vi "Choose case dewbot 10.vi"(4 "Next FR motor value":dbl=0.6, 6 "Next BL motor value":dbl=0.6, 9 "Next BR motor value":dbl=0.6, 10 "Next FL motor value":dbl=0.6, 11 "Set Tac value":dbl) -> (0 "Last FR motor value":dbl=0.6, 1 "Last BL motor value":dbl=0.6, 2 "Last BR motor value":dbl=0.6, 3 "Last FL motor value":dbl=0.6, 5 "Next primitive?":bool)   [LabVIEW 2013]
uses:
  Begin/Global Variables.vi
  Begin/Global Refnums.vi
  <vilib>/Rock Robotics/WPI/DriverStation/DriverStationLCD/WPI_DriverStationLCDLCDLine.ctl
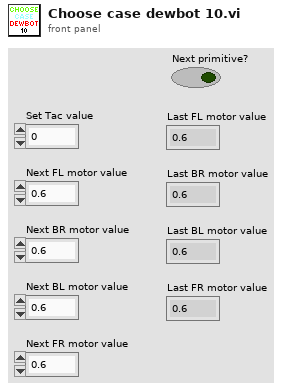
[diagram p1: front panel]
types:
  T1 = typedef "WPI_DriverStationLCDLCDLine.ctl" = enum16{"Main - Line 1", "User - Line 2", "User - Line 3", "User - Line 4", "User - Line 5", "User - Line 6"}
  T2 = typedef "WPI_GyroDevRef.ctl" = cluster{"DevStatus":errorcluster, "Analog Module":T3, "Analog Channel":T4, "Offset":dbl, "Gain (VoltsPerDegree/Second)":dbl}
  T3 = typedef "FPGA_TypedefAnalogModule.ctl" = enum16{"Analog Module 1", "Analog Module 2"}
  T4 = typedef "FPGA_AIChannel.ctl" = enum8{"AI 1", "AI 2", "AI 3", "AI 4", "AI 5", "AI 6", "AI 7", "AI 8", "Invalid"}
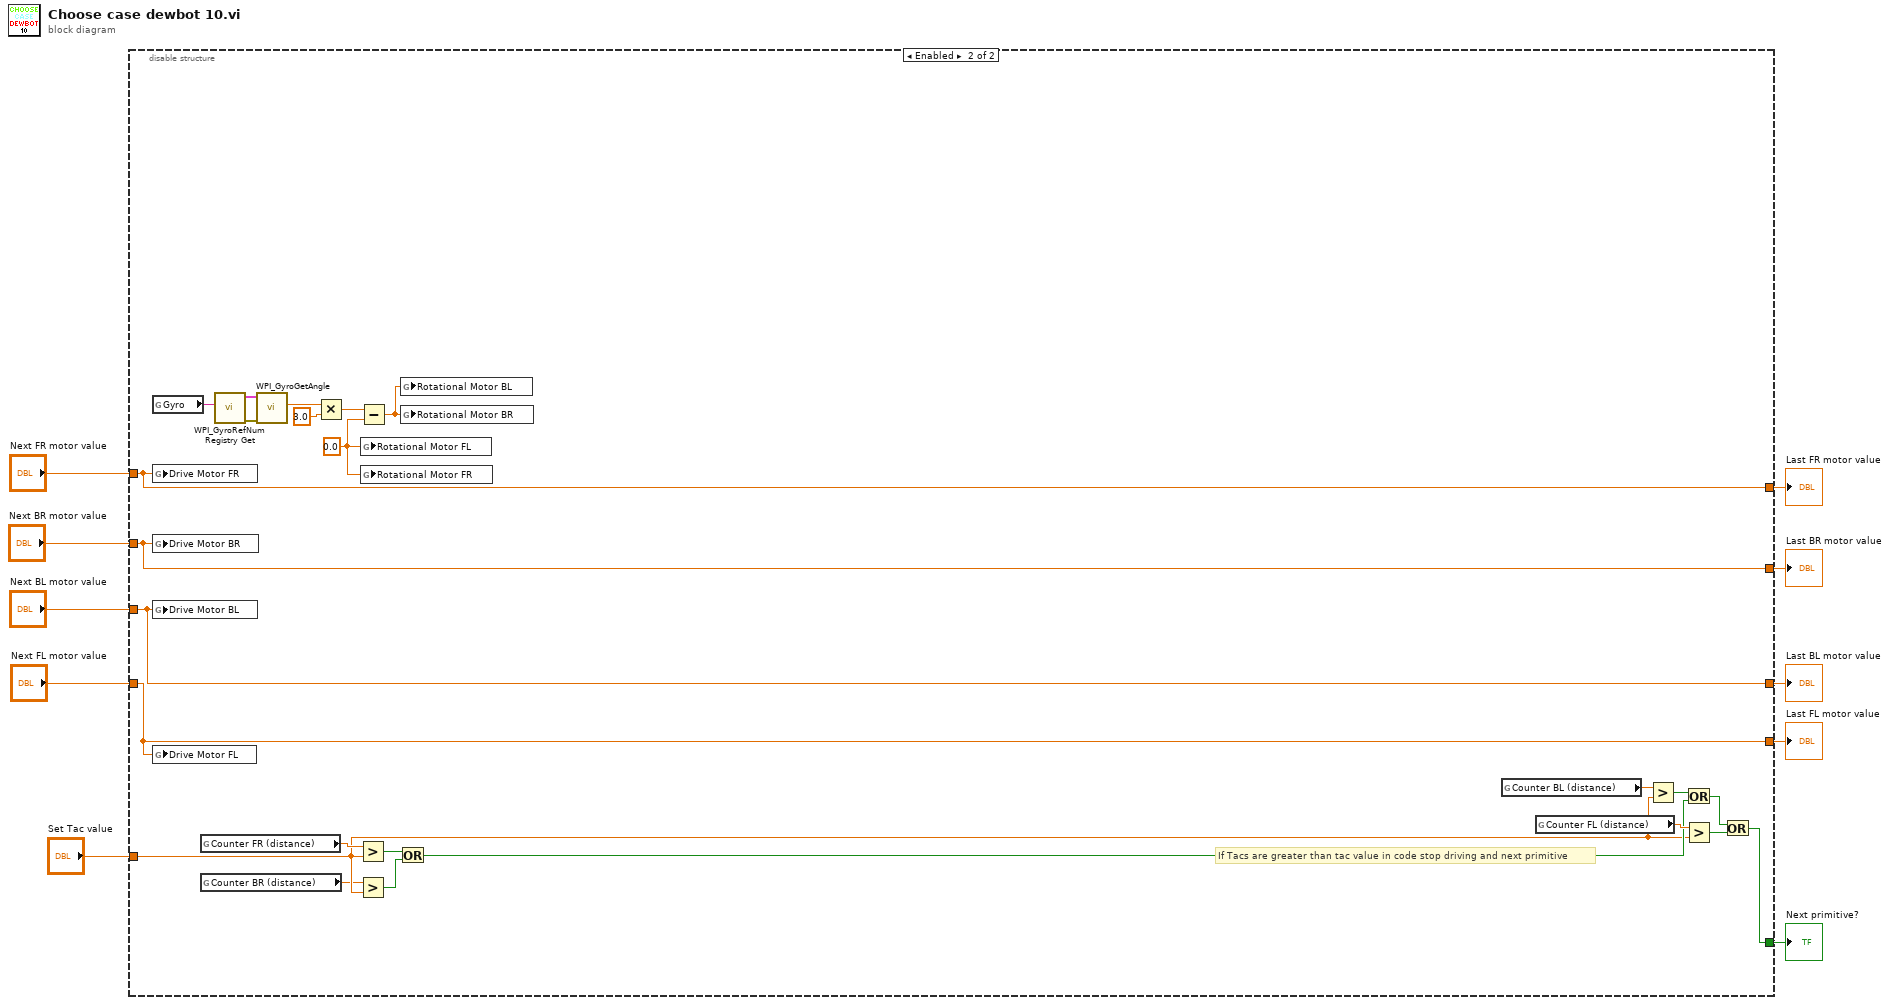
[diagram p0: block diagram]
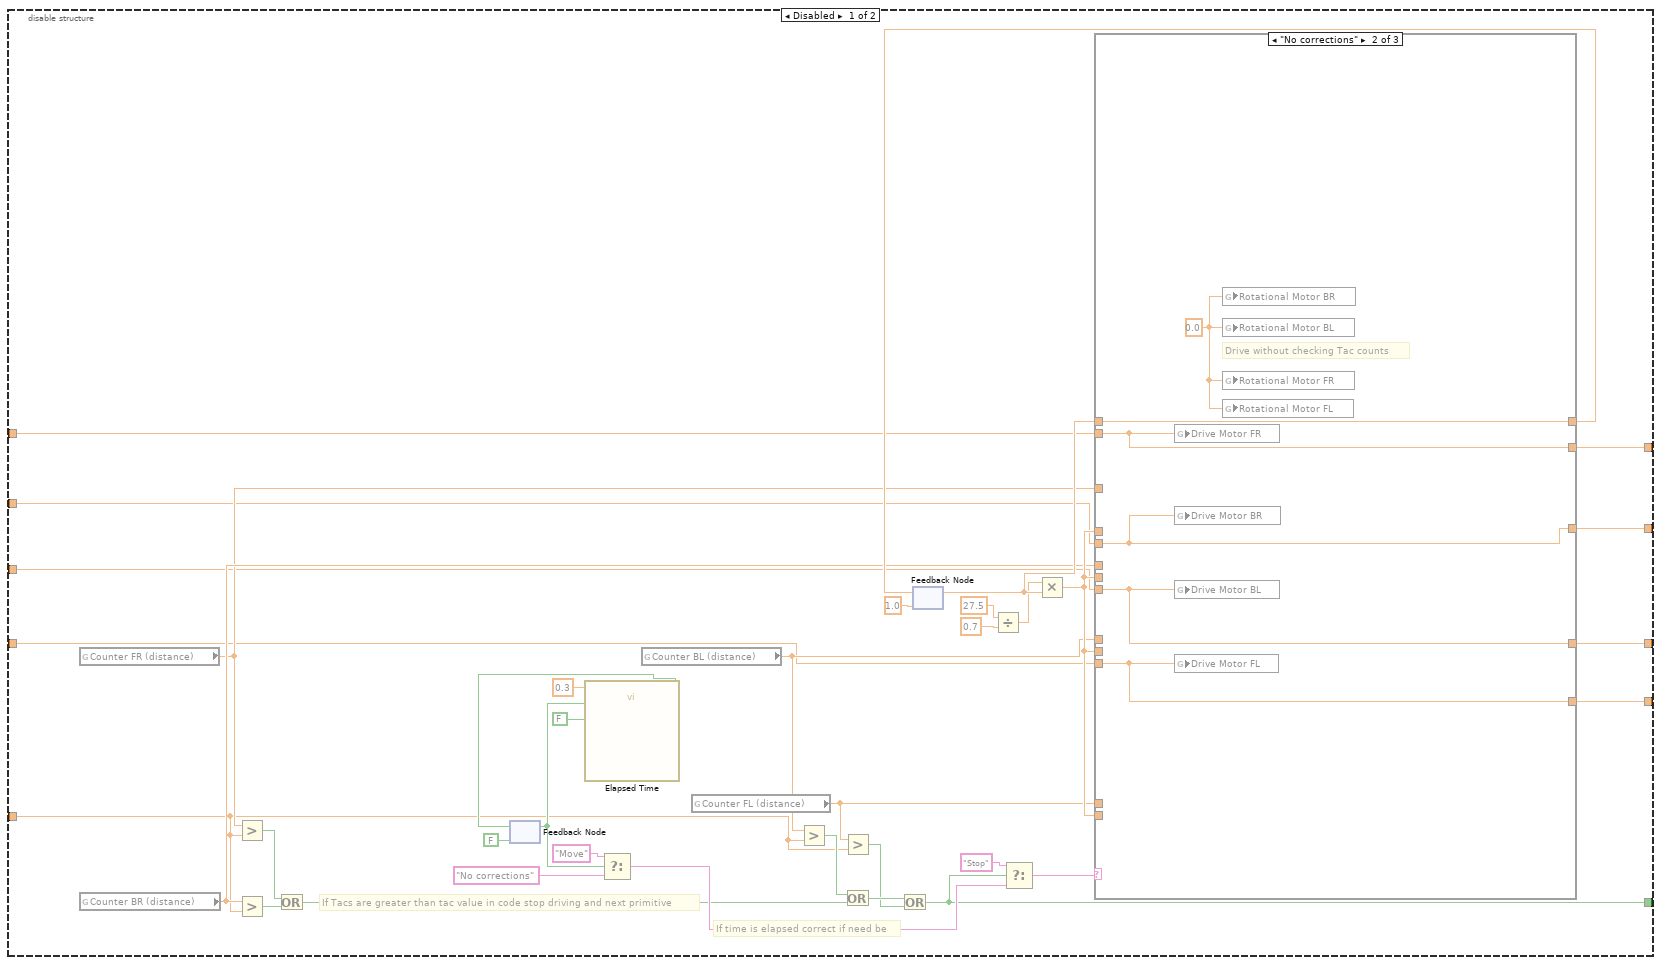
[diagram p2: hidden frame]
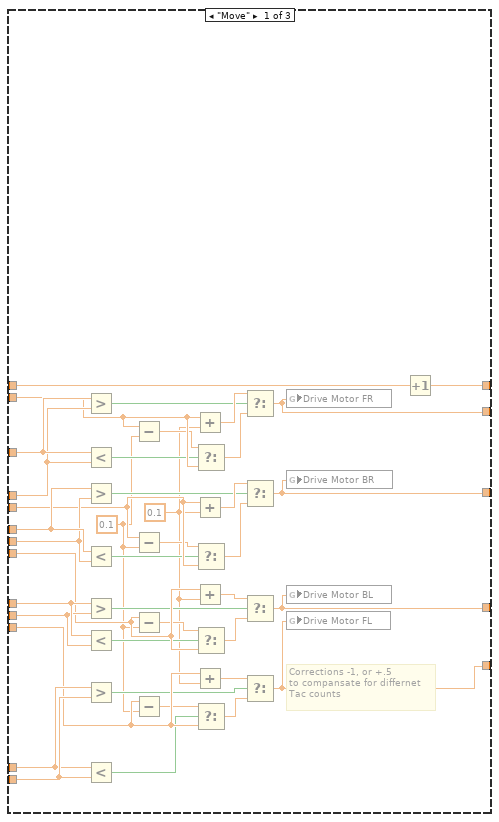
[diagram p3: hidden frame]
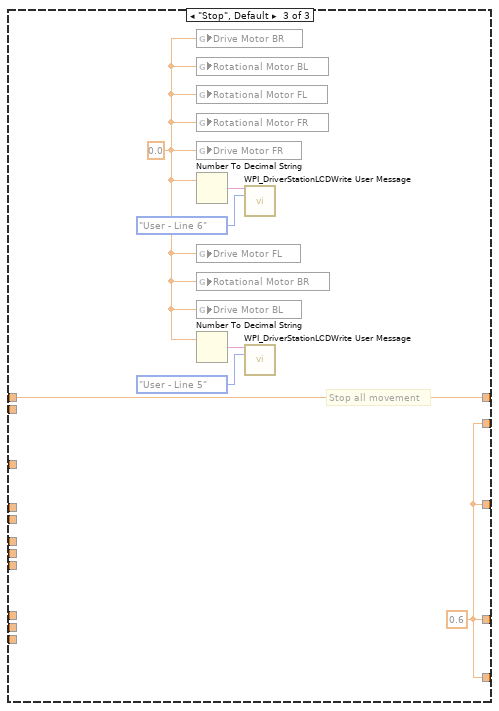
[diagram p4: hidden frame]
diagram:
  n1 = disable-structure shown="Enabled" {
    disable-tunnel: "Set Tac value" -> [w20 w114]
    disable-tunnel: [w19 w115] -> w9
    disable-tunnel: "Next BR motor value" -> [w18 w112]
    disable-tunnel: "Next FR motor value" -> [w17 w110]
    disable-tunnel: "Next BL motor value" -> [w16 w109]
    disable-tunnel: "Next FL motor value" -> [w15 w111]
    disable-tunnel: [w14 w112] -> w4
    disable-tunnel: [w13 w111] -> w3
    disable-tunnel: [w12 w110] -> w2
    disable-tunnel: [w11 w109] -> w1
    frame Disabled {
      # "If time is elapsed correct if need be"
      # "If Tacs are greater than tac value in code stop driving and next primitive"
      n2 = global read "Global Refnums.vi" "Counter FR (distance)"() -> (w25:dbl)
      n3 = global read "Global Refnums.vi" "Counter BR (distance)"() -> (w27:dbl)
      n4 = Greater?(x=w25, y=w20) -> (0:w38:bool)
      n5 = Greater?(x=w27, y=w20) -> (0:w39:bool)
      n6 = Or(x=w38, y=w39) -> (x .or. y?=w24:bool)
      n7 = feedback #1(FALSE ("Time has Elapsed")) -> (w30:bool)
      n8 = call "Elapsed Time"("Time Target (s)"=0.3, "Reset"=w30, "Auto Reset"=FALSE) -> ("Time has Elapsed"=w31:bool)  [unwired: 9 in, 7 out]
      n9 = feedback-in #1(w31) -> ()
      n10 = Select(t="Move" ("f"), s=w30, f="No corrections" ("t")) -> (s? t:f=w32:string)
      n11 = global read "Global Refnums.vi" "Counter BL (distance)"() -> (w28:dbl)
      n12 = global read "Global Refnums.vi" "Counter FL (distance)"() -> (w26:dbl)
      n13 = Greater?(x=w28, y=w20) -> (0:w37:bool)
      n14 = Greater?(x=w26, y=w20) -> (0:w23:bool)
      n15 = Or(x=w37, y=w24) -> (x .or. y?=w36:bool)
      n16 = Or(x=w36, y=w23) -> (x .or. y?=w19:bool)
      n17 = feedback #2(1.0) -> (w47:dbl)
      n18 = Divide(x=27.5, y=0.7) -> (x/y=w21:dbl)
      n19 = Select(t="Stop", s=w19, f=w32) -> (s? t:f=w34:string)
      n20 = Multiply(x=w21, y=w47) -> (x*y=w45:dbl)
      n21 = case shown="\"No corrections\"" w34 {
        tunnel: [w84 w90 w95] -> w12
        tunnel: w16 -> [w76 w92 _]
        tunnel: w27 -> [w87 _ _]
        tunnel: w25 -> [w86 _ _]
        tunnel: w26 -> [w73 _ _]
        tunnel: w28 -> [w85 _ _]
        tunnel: [w83 w91 w95] -> w13
        tunnel: [w82 w92 w95] -> w11
        tunnel: [w81 w93 w95] -> w14
        tunnel: w17 -> [w74 w90 _]
        tunnel: w18 -> [w75 w93 _]
        tunnel: w15 -> [w72 w91 _]
        tunnel: w45 -> [w80 _ _]
        tunnel: w45 -> [w79 _ _]
        tunnel: w45 -> [w78 _ _]
        tunnel: w45 -> [w77 _ _]
        tunnel: [w71 w88 w94] -> w42
        tunnel: w47 -> [w70 w88 w94]
        frame "Move" {
          w48 = 0.1 ("Time Target (s)")
          w49 = 0.1 ("Time Target (s)")
          # "Corrections -1, or +.5 \nto compansate for differnet\nTac counts"
          n22 = Greater?(x=w86, y=w80) -> (0:w60:bool)
          n23 = Less?(x=w86, y=w80) -> (x < y?=w61:bool)
          n24 = Greater?(x=w87, y=w79) -> (0:w66:bool)
          n25 = Less?(x=w87, y=w79) -> (x < y?=w65:bool)
          n26 = Greater?(x=w85, y=w78) -> (0:w50:bool)
          n27 = Less?(x=w85, y=w78) -> (x < y?=w51:bool)
          n28 = Greater?(x=w73, y=w77) -> (0:w55:bool)
          n29 = Less?(x=w73, y=w77) -> (x < y?=w56:bool)
          n30 = Subtract(x=w74, y=w48) -> (x-y=w63:dbl)
          n31 = Subtract(x=w75, y=w48) -> (x-y=w68:dbl)
          n32 = Subtract(x=w76, y=w48) -> (x-y=w53:dbl)
          n33 = Subtract(x=w72, y=w48) -> (x-y=w59:dbl)
          n34 = Add(x=w74, y=w49) -> (x+y=w64:dbl)
          n35 = Add(x=w75, y=w49) -> (x+y=w69:dbl)
          n36 = Add(x=w76, y=w49) -> (x+y=w54:dbl)
          n37 = Add(x=w72, y=w49) -> (x+y=w58:dbl)
          n38 = Select(t=w63, s=w61, f=w74) -> (s? t:f=w62:dbl)
          n39 = Select(t=w68, s=w65, f=w75) -> (s? t:f=w67:dbl)
          n40 = Select(t=w53, s=w51, f=w76) -> (s? t:f=w52:dbl)
          n41 = Select(t=w59, s=w56, f=w72) -> (s? t:f=w57:dbl)
          n42 = Select(t=w64, s=w60, f=w62) -> (s? t:f=w84:dbl)
          n43 = Select(t=w69, s=w66, f=w67) -> (s? t:f=w81:dbl)
          n44 = Select(t=w54, s=w50, f=w52) -> (s? t:f=w82:dbl)
          n45 = Select(t=w58, s=w55, f=w57) -> (s? t:f=w83:dbl)
          n46 = global write "Global Variables.vi" "Drive Motor FR"(w84) -> ()
          n47 = global write "Global Variables.vi" "Drive Motor BR"(w81) -> ()
          n48 = global write "Global Variables.vi" "Drive Motor BL"(w82) -> ()
          n49 = global write "Global Variables.vi" "Drive Motor FL"(w83) -> ()
          n50 = Increment(x=w70) -> (x+1=w71:dbl)
        }
        frame "No corrections" {
          w89 = 0.0
          # "Drive without checking Tac counts"
          n51 = global write "Global Variables.vi" "Drive Motor FR"(w90) -> ()
          n52 = global write "Global Variables.vi" "Drive Motor BR"(w93) -> ()
          n53 = global write "Global Variables.vi" "Drive Motor BL"(w92) -> ()
          n54 = global write "Global Variables.vi" "Drive Motor FL"(w91) -> ()
          n55 = global write "Global Variables.vi" "Rotational Motor BR"(w89) -> ()
          n56 = global write "Global Variables.vi" "Rotational Motor BL"(w89) -> ()
          n57 = global write "Global Variables.vi" "Rotational Motor FR"(w89) -> ()
          n58 = global write "Global Variables.vi" "Rotational Motor FL"(w89) -> ()
        }
        frame "Stop", Default {
          w95 = 0.6 ("upper limit")
          w96 = 0.0
          # "Stop all movement"
          n59 = global write "Global Variables.vi" "Drive Motor BR"(w96) -> ()
          n60 = global write "Global Variables.vi" "Rotational Motor BL"(w96) -> ()
          n61 = global write "Global Variables.vi" "Rotational Motor FL"(w96) -> ()
          n62 = global write "Global Variables.vi" "Rotational Motor FR"(w96) -> ()
          n63 = global write "Global Variables.vi" "Drive Motor FR"(w96) -> ()
          n64 = Number To Decimal String(number=w96) -> (decimal integer string=w99:string)  [unwired: 1 in]
          n65 = global write "Global Variables.vi" "Drive Motor FL"(w96) -> ()
          n66 = global write "Global Variables.vi" "Rotational Motor BR"(w96) -> ()
          n67 = global write "Global Variables.vi" "Drive Motor BL"(w96) -> ()
          n68 = Number To Decimal String(number=w96) -> (decimal integer string=w100:string)  [unwired: 1 in]
          n69 = call <vilib>:"WPI_DriverStationLCDWrite User Message.vi"("line text"=w99, "line"=WPI_DriverStationLCDLCDLine."User - Line 6") -> ()  [unwired: 13 in, 1 out]
          n70 = call <vilib>:"WPI_DriverStationLCDWrite User Message.vi"("line text"=w100, "line"=WPI_DriverStationLCDLCDLine."User - Line 5") -> ()  [unwired: 13 in, 1 out]
        }
      }
      n71 = feedback-in #2(w42) -> ()
    }
    frame Enabled {
      w101 = 0.0 ("t")
      # "If Tacs are greater than tac value in code stop driving and next primitive"
      n72 = global read "Global Refnums.vi" "Gyro"() -> (w102:string)
      n73 = global write "Global Variables.vi" "Drive Motor FR"(w110) -> ()
      n74 = global write "Global Variables.vi" "Drive Motor BR"(w112) -> ()
      n75 = global write "Global Variables.vi" "Drive Motor BL"(w109) -> ()
      n76 = global write "Global Variables.vi" "Drive Motor FL"(w111) -> ()
      n77 = global read "Global Refnums.vi" "Counter FR (distance)"() -> (w118:dbl)
      n78 = global read "Global Refnums.vi" "Counter BR (distance)"() -> (w113:dbl)
      n79 = call <vilib>:"WPI_GyroRefNum Registry Get.vi"("refnum name"=w102) -> ("error out"=w107:errorcluster, "GyroDevRef"=w106:T2)  [unwired: 9 in]
      n80 = call <vilib>:"WPI_GyroGetAngle.vi"("error in (no error)"=w107, "GyroDevRef"=w106) -> ("Angle"=w105:dbl)  [unwired: 6 in, 3 out]
      n81 = Multiply(x=w105, y=3.0) -> (x*y=w103:dbl)
      n82 = Greater?(x=w118, y=w114) -> (0:w123:bool)
      n83 = Greater?(x=w113, y=w114) -> (0:w124:bool)
      n84 = Subtract(x=w103, y=w101) -> (x-y=w108:dbl)
      n85 = global write "Global Variables.vi" "Rotational Motor FL"(w101) -> ()
      n86 = global write "Global Variables.vi" "Rotational Motor FR"(w101) -> ()
      n87 = Or(x=w123, y=w124) -> (x .or. y?=w117:bool)
      n88 = global write "Global Variables.vi" "Rotational Motor BL"(w108) -> ()
      n89 = global write "Global Variables.vi" "Rotational Motor BR"(w108) -> ()
      n90 = global read "Global Refnums.vi" "Counter BL (distance)"() -> (w120:dbl)
      n91 = global read "Global Refnums.vi" "Counter FL (distance)"() -> (w119:dbl)
      n92 = Greater?(x=w120, y=w114) -> (0:w122:bool)
      n93 = Or(x=w122, y=w117) -> (x .or. y?=w121:bool)
      n94 = Greater?(x=w119, y=w114) -> (0:w116:bool)
      n95 = Or(x=w121, y=w116) -> (x .or. y?=w115:bool)
    }
  }
  "Next primitive?" <- w9
  "Last BR motor value" <- w4
  "Last FL motor value" <- w3
  "Last FR motor value" <- w2
  "Last BL motor value" <- w1
